vi "ProjectClassVI.vi"(11 "Color Box":u32(colorbox)=16918) -> (3 "Color/2":dbl=7790.0)   [LabVIEW 2023, in "ProjectClass.lvclass"]
doc: "Input = Blue color [15580]\nOutput = Color/2"
uses:
  ProjectClass.lvclass
panel:
  out "Numeric":dbl=15580.0
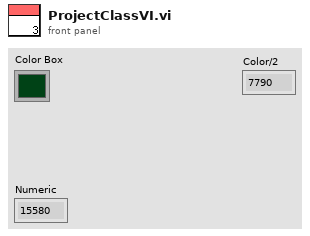
[diagram p1: front panel]
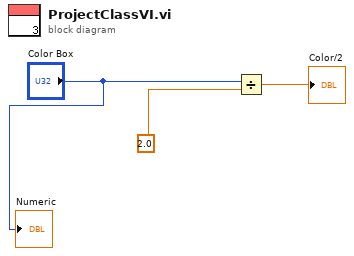
[diagram p0: block diagram]
diagram:
  n1 = Divide(x="Color Box", y=2.0) -> (x/y=→"Color/2":dbl)
  "Numeric" <- "Color Box"
